vi "Disable.vi"   [LabVIEW 2016]
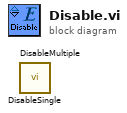
[diagram p0: block diagram]
diagram:
  n1 = call "DisableMultiple.vi"() -> ()  [unwired: 10 in, 2 out]
  n2 = call "DisableSingle.vi"() -> ()  [unwired: 10 in, 2 out]
